vi "PGSQL.Open.vi"(8 "error in (no error)":errorcluster, 10 "Connection String":string, 11 "Data.PG in":refnum<class "LV-Data.PGSQL.lvclass">) -> (0 "error out":errorcluster, 3 "Data.PG out":refnum<class "LV-Data.PGSQL.lvclass">)   [LabVIEW 2019, in "LV-Data.PGSQL.lvclass"]
uses:
  LV-Data.PGSQL.lvclass
  LV-Data.PGSQL.lvclass/LV-Data.PGSQL.ctl
  <vilib>/JDP Science/PostgreSQL Library/Connection/PQ Connection.lvclass
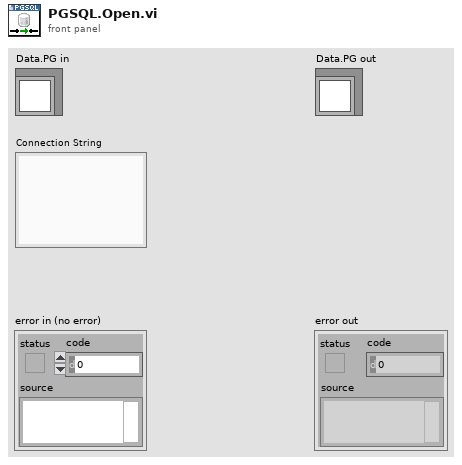
[diagram p1: front panel]
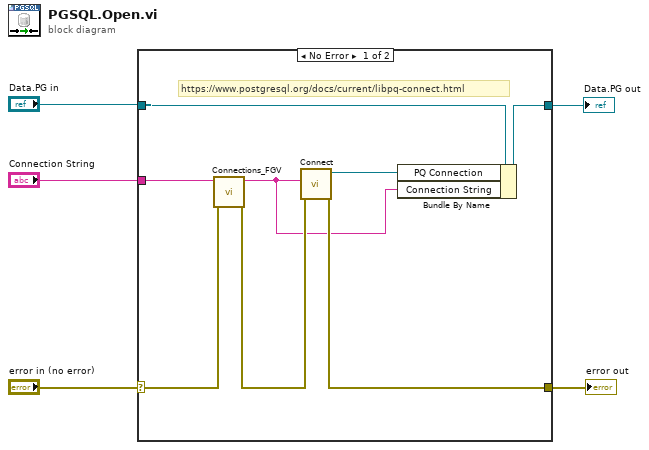
[diagram p0: block diagram]
diagram:
  n1 = case shown="No Error" "error in (no error)" {
    selector: "error in (no error)" -> [w10 w15]
    tunnel: [w7 w15] -> w5
    tunnel: "Data.PG in" -> [w11 w14]
    tunnel: [w13 w14] -> w4
    tunnel: "Connection String" -> [w9 _]
    frame No Error {
      # "https://www.postgresql.org/docs/current/libpq-connect.html"
      n2 = call "Connections_FGV.vi"("error in (no error)"=w10, "connection string in"=w9) -> ("error out"=w8:errorcluster, "connection string out"=w6:string)  [unwired: 8 in]
      n3 = call <vilib>:"Connect.vi"("error in (no error)"=w8, "Connection Strings"=w6) -> ("error out"=w7:errorcluster, "PQ Connection"=w12:refnum<class "PQ Connection.lvclass">)  [unwired: 8 in]
      n4 = Bundle By Name(cluster=w11, "PQ Connection"=w12, "Connection String"=w6) -> (w13:refnum<class "LV-Data.PGSQL.lvclass">)
    }
    frame Error {
    }
  }
  "error out" <- w5
  "Data.PG out" <- w4
